vi "Test Case Runner.vi"(0 "Problem":T1, 1 "Numeric 2":dbl, 2 "Numeric Array 2":dbl[](array[numeric]), 3 "String 2":string, 4 "String Array 2":string[](array[string]), 5 "Iterator":i32, 8 "TestCases Folder":path, 9 "Send Input?":bool) -> (15 "Numeric":dbl, 16 "Numeric Array":dbl[](array[numeric]), 17 "String":string, 18 "String Array":string[](array[string]), 19 "Accepted":bool)   [LabVIEW 2014]
uses:
  Main Contest/Problem.ctl
  <vilib>/Utility/file.llb/Read From Spreadsheet File (string).vi
  <vilib>/Utility/file.llb/Read From Spreadsheet File (DBL).vi
panel:
  out "E":path=path "C:/Users/Justin/Desktop/LabVIEW-Rank/Offline Judge/TestCases/Test A.csv"
  out "D":path=path "C:/Users/Justin/Desktop/LabVIEW-Rank/Offline Judge/TestCases/Test A.csv"
  out "C":path=path "C:/Users/Justin/Desktop/LabVIEW-Rank/Offline Judge/TestCases/Test A.csv"
  out "B":path=path "C:/Users/Justin/Desktop/LabVIEW-Rank/Offline Judge/TestCases/Test A.csv"
  out "A":path=path "C:/Users/Justin/Desktop/LabVIEW-Rank/Offline Judge/TestCases/Test A.csv"
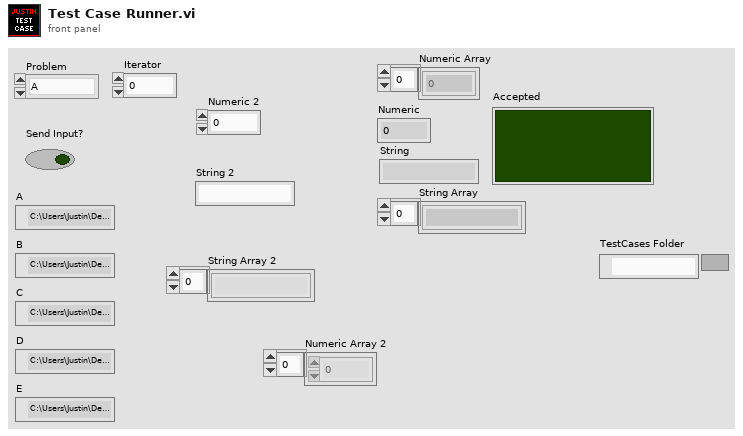
[diagram p1: front panel]
types:
  T1 = typedef "Problem.ctl" = enum16{"A", "B", "C", "D", "E"}
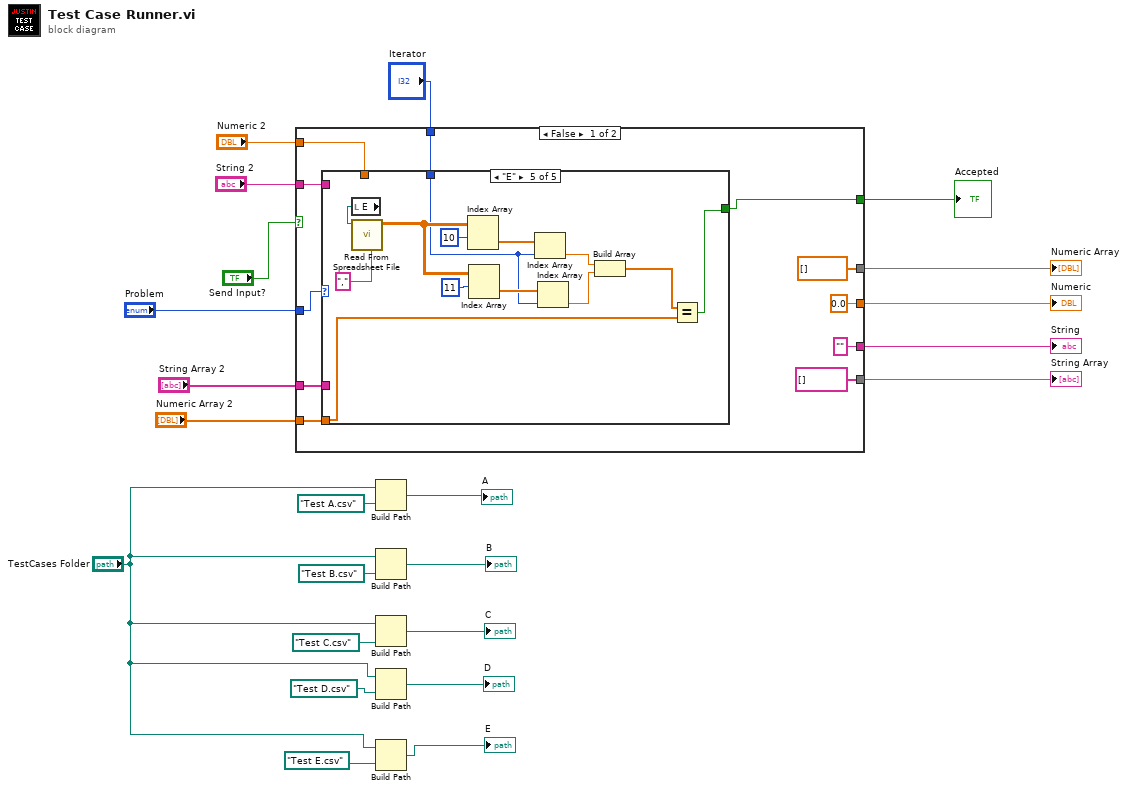
[diagram p0: block diagram]
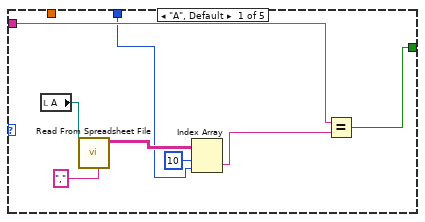
[diagram p2: hidden frame]
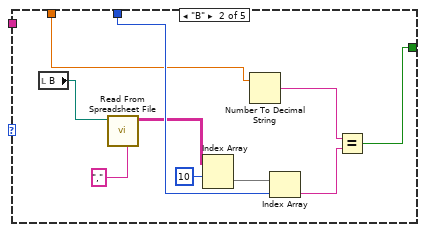
[diagram p3: hidden frame]
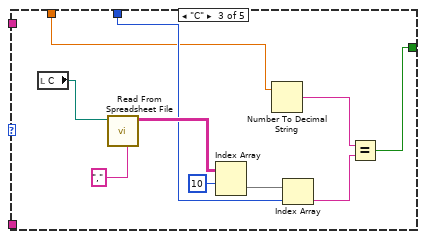
[diagram p4: hidden frame]
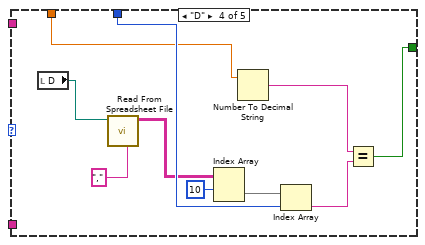
[diagram p5: hidden frame]
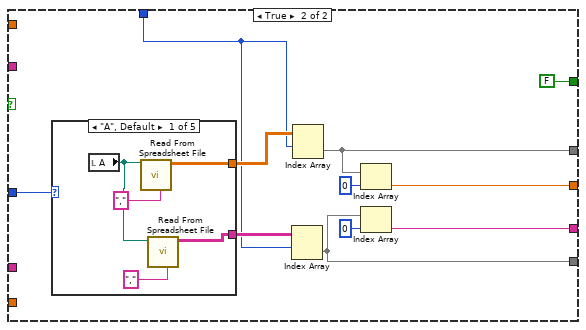
[diagram p6: hidden frame]
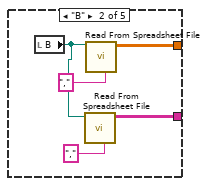
[diagram p7: hidden frame]
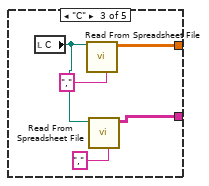
[diagram p8: hidden frame]
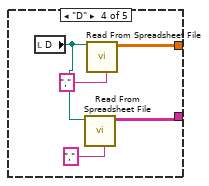
[diagram p9: hidden frame]
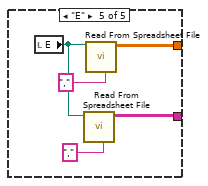
[diagram p10: hidden frame]
diagram:
  n1 = case shown="False" "Send Input?" {
    tunnel: "Problem" -> [w34 w96]
    tunnel: [w24 FALSE] -> w21
    tunnel: "Iterator" -> [w25 w89]
    tunnel: [dbl[] [] ("all rows") w93] -> w19
    tunnel: [0.0 w91] -> w18
    tunnel: [string[] [] ("all rows") w87] -> w16
    tunnel: ["" ("String") w86] -> w17
    tunnel: "Numeric 2" -> [w29 _]
    tunnel: "String Array 2" -> [w28 _]
    tunnel: "Numeric Array 2" -> [w27 _]
    tunnel: "String 2" -> [w26 _]
    frame False {
      n2 = case shown="\"E\"" w34 {
        tunnel: w29 -> [_ w45 w55 w63 _]
        tunnel: w28 -> [_ _ _ _ _]
        tunnel: w27 -> [_ _ _ _ w73]
        tunnel: w26 -> [w38 _ _ _ _]
        tunnel: w25 -> [w37 w48 w57 w68 w77]
        tunnel: [w39 w46 w56 w66 w82] -> w24
        frame "A", Default {
          n3 = local read "A"() -> (w42:path)
          n4 = call-poly <vilib>:"Read From Spreadsheet File.vi"("delimiter (\\t)"="," ("delimiter (\\t)"), "file path (dialog if empty)"=w42) -> ("all rows"=w41:string[][])  [unwired: 5 in, 4 out]
          n5 = Index Array(array=w41, index (row)=10, index (col)=w37) -> (element=w36:string)
          n6 = Equal?(x=w38, y=w36) -> (x = y?=w39:bool)
        }
        frame "B" {
          n7 = local read "B"() -> (w52:path)
          n8 = call-poly <vilib>:"Read From Spreadsheet File.vi"("delimiter (\\t)"="," ("delimiter (\\t)"), "file path (dialog if empty)"=w52) -> ("all rows"=w47:string[][])  [unwired: 5 in, 4 out]
          n9 = Index Array(array=w47, index (row)=10) -> (element=w50:string[])  [unwired: 1 in]
          n10 = Number To Decimal String(number=w45) -> (decimal integer string=w44:string)  [unwired: 1 in]
          n11 = Index Array(array=w50, index=w48) -> (element=w51:string)
          n12 = Equal?(x=w44, y=w51) -> (x = y?=w46:bool)
        }
        frame "C" {
          n13 = local read "C"() -> (w62:path)
          n14 = call-poly <vilib>:"Read From Spreadsheet File.vi"("delimiter (\\t)"="," ("delimiter (\\t)"), "file path (dialog if empty)"=w62) -> ("all rows"=w58:string[][])  [unwired: 5 in, 4 out]
          n15 = Index Array(array=w58, index (row)=10) -> (element=w60:string[])  [unwired: 1 in]
          n16 = Number To Decimal String(number=w55) -> (decimal integer string=w54:string)  [unwired: 1 in]
          n17 = Index Array(array=w60, index=w57) -> (element=w61:string)
          n18 = Equal?(x=w54, y=w61) -> (x = y?=w56:bool)
        }
        frame "D" {
          n19 = local read "D"() -> (w72:path)
          n20 = call-poly <vilib>:"Read From Spreadsheet File.vi"("delimiter (\\t)"="," ("delimiter (\\t)"), "file path (dialog if empty)"=w72) -> ("all rows"=w67:string[][])  [unwired: 5 in, 4 out]
          n21 = Index Array(array=w67, index (row)=10) -> (element=w70:string[])  [unwired: 1 in]
          n22 = Number To Decimal String(number=w63) -> (decimal integer string=w64:string)  [unwired: 1 in]
          n23 = Index Array(array=w70, index=w68) -> (element=w69:string)
          n24 = Equal?(x=w64, y=w69) -> (x = y?=w66:bool)
        }
        frame "E" {
          n25 = local read "E"() -> (w85:path)
          n26 = call-poly <vilib>:"Read From Spreadsheet File.vi"("delimiter (\\t)"="," ("delimiter (\\t)"), "file path (dialog if empty)"=w85) -> ("all rows"=w79:dbl[][])  [unwired: 5 in, 4 out]
          n27 = Index Array(array=w79, index (row)=10) -> (element=w83:dbl[])  [unwired: 1 in]
          n28 = Index Array(array=w79, index (row)=11) -> (element=w78:dbl[])  [unwired: 1 in]
          n29 = Index Array(array=w83, index=w77) -> (element=w76:dbl)
          n30 = Index Array(array=w78, index=w77) -> (element=w75:dbl)
          n31 = Build Array(w76, w75) -> (w74:dbl[])
          n32 = Equal?(x=w74, y=w73) -> (x = y?=w82:bool)
        }
      }
    }
    frame True {
      n33 = case shown="\"A\", Default" w96 {
        tunnel: [w100 w106 w109 w115 w119] -> w94
        tunnel: [w99 w104 w110 w116 w120] -> w90
        frame "A", Default {
          n34 = local read "A"() -> (w101:path)
          n35 = call-poly <vilib>:"Read From Spreadsheet File.vi"("delimiter (\\t)"="," ("delimiter (\\t)"), "file path (dialog if empty)"=w101) -> ("all rows"=w100:dbl[][])  [unwired: 5 in, 4 out]
          n36 = call-poly <vilib>:"Read From Spreadsheet File.vi"("delimiter (\\t)"="," ("delimiter (\\t)"), "file path (dialog if empty)"=w101) -> ("all rows"=w99:string[][])  [unwired: 5 in, 4 out]
        }
        frame "B" {
          n37 = local read "B"() -> (w105:path)
          n38 = call-poly <vilib>:"Read From Spreadsheet File.vi"("delimiter (\\t)"="," ("delimiter (\\t)"), "file path (dialog if empty)"=w105) -> ("all rows"=w104:string[][])  [unwired: 5 in, 4 out]
          n39 = call-poly <vilib>:"Read From Spreadsheet File.vi"("delimiter (\\t)"="," ("delimiter (\\t)"), "file path (dialog if empty)"=w105) -> ("all rows"=w106:dbl[][])  [unwired: 5 in, 4 out]
        }
        frame "C" {
          n40 = local read "C"() -> (w111:path)
          n41 = call-poly <vilib>:"Read From Spreadsheet File.vi"("delimiter (\\t)"="," ("delimiter (\\t)"), "file path (dialog if empty)"=w111) -> ("all rows"=w109:dbl[][])  [unwired: 5 in, 4 out]
          n42 = call-poly <vilib>:"Read From Spreadsheet File.vi"("delimiter (\\t)"="," ("delimiter (\\t)"), "file path (dialog if empty)"=w111) -> ("all rows"=w110:string[][])  [unwired: 5 in, 4 out]
        }
        frame "D" {
          n43 = local read "D"() -> (w114:path)
          n44 = call-poly <vilib>:"Read From Spreadsheet File.vi"("delimiter (\\t)"="," ("delimiter (\\t)"), "file path (dialog if empty)"=w114) -> ("all rows"=w116:string[][])  [unwired: 5 in, 4 out]
          n45 = call-poly <vilib>:"Read From Spreadsheet File.vi"("delimiter (\\t)"="," ("delimiter (\\t)"), "file path (dialog if empty)"=w114) -> ("all rows"=w115:dbl[][])  [unwired: 5 in, 4 out]
        }
        frame "E" {
          n46 = local read "E"() -> (w121:path)
          n47 = call-poly <vilib>:"Read From Spreadsheet File.vi"("delimiter (\\t)"="," ("delimiter (\\t)"), "file path (dialog if empty)"=w121) -> ("all rows"=w120:string[][])  [unwired: 5 in, 4 out]
          n48 = call-poly <vilib>:"Read From Spreadsheet File.vi"("delimiter (\\t)"="," ("delimiter (\\t)"), "file path (dialog if empty)"=w121) -> ("all rows"=w119:dbl[][])  [unwired: 5 in, 4 out]
        }
      }
      n49 = Index Array(array=w90, index (row)=w89) -> (element=w87:string[])  [unwired: 1 in]
      n50 = Index Array(array=w94, index (row)=w89) -> (element=w93:dbl[])  [unwired: 1 in]
      n51 = Index Array(array=w93, index=0) -> (element=w91:dbl)
      n52 = Index Array(array=w87, index=0) -> (element=w86:string)
    }
  }
  "Accepted" <- w21
  "Numeric Array" <- w19
  "Numeric" <- w18
  "String" <- w17
  "String Array" <- w16
  n53 = Build Path(base path="TestCases Folder", name or relative path=path "Test A.csv" ("file path (dialog if empty)")) -> (appended path=→"A":path)
  n54 = Build Path(base path="TestCases Folder", name or relative path=path "Test B.csv" ("file path (dialog if empty)")) -> (appended path=→"B":path)
  n55 = Build Path(base path="TestCases Folder", name or relative path=path "Test C.csv" ("file path (dialog if empty)")) -> (appended path=→"C":path)
  n56 = Build Path(base path="TestCases Folder", name or relative path=path "Test D.csv" ("file path (dialog if empty)")) -> (appended path=→"D":path)
  n57 = Build Path(base path="TestCases Folder", name or relative path=path "Test E.csv" ("file path (dialog if empty)")) -> (appended path=→"E":path)
